vi "Start.vi"(8 "error in (no error)":errorcluster, 10 "Message in":refnum<class "StartMessage.lvclass">, 11 "DAQMH121119OrcaFlash in":refnum<class "DAQOrcaFlash.lvclass">) -> (0 "error out":errorcluster, 3 "DAQMH121119OrcaFlash out":refnum<class "DAQOrcaFlash.lvclass">)   [LabVIEW 2012, in "DAQOrcaFlash.lvclass"]
doc: "This member function is called when the statemachine in the run.vi receives an 'start' command. It relays the message to all observers of the component.\n\nOverride this member function in your derived class if you need additional start functionality (but don't forget to call the parent method)."
uses:
  DAQOrcaFlash.lvclass
  <vilib>/Distrio/Murmex/StartMessage/StartMessage.lvclass
  <vilib>/Distrio/Murmex/Murmex/Murmex.lvclass
  DAQOrcaFlash.lvclass/DAQOrcaFlash.ctl
  <vilib>/Distrio/Murmex/ProceedMessage/ProceedMessage.lvclass
  imaging_mode.ctl
panel:
  # "This method is called when the START\ntrigger is sent. \n\nOverride this method when your component needs to\nrespond to this trigger. \n\nCall parent for proper implementation"
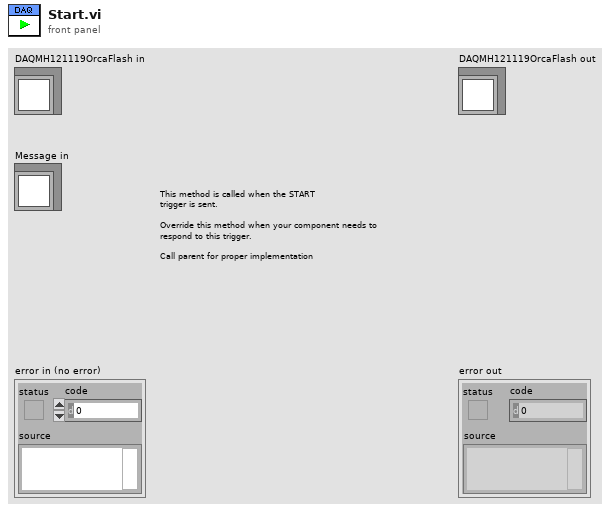
[diagram p1: front panel]
types:
  T1 = cluster{"Mode":u32, "Polarity":u32, "Period":dbl, "Delay":dbl}
  T2 = typedef "DAQOrcaFlash.lvclass/imaging_mode.ctl" = enum16{"focus mode", "single sweep"}
  T3 = typedef "Murmex.lvlib/StartMessage.lvclass/run mode enum.ctl" = enum16{"infinite", "finite"}
  T4 = typedef "IMAQ Image.ctl" = refnum<image>
  T5 = cluster{"width":u32, "height":u32, "datatype":u32}
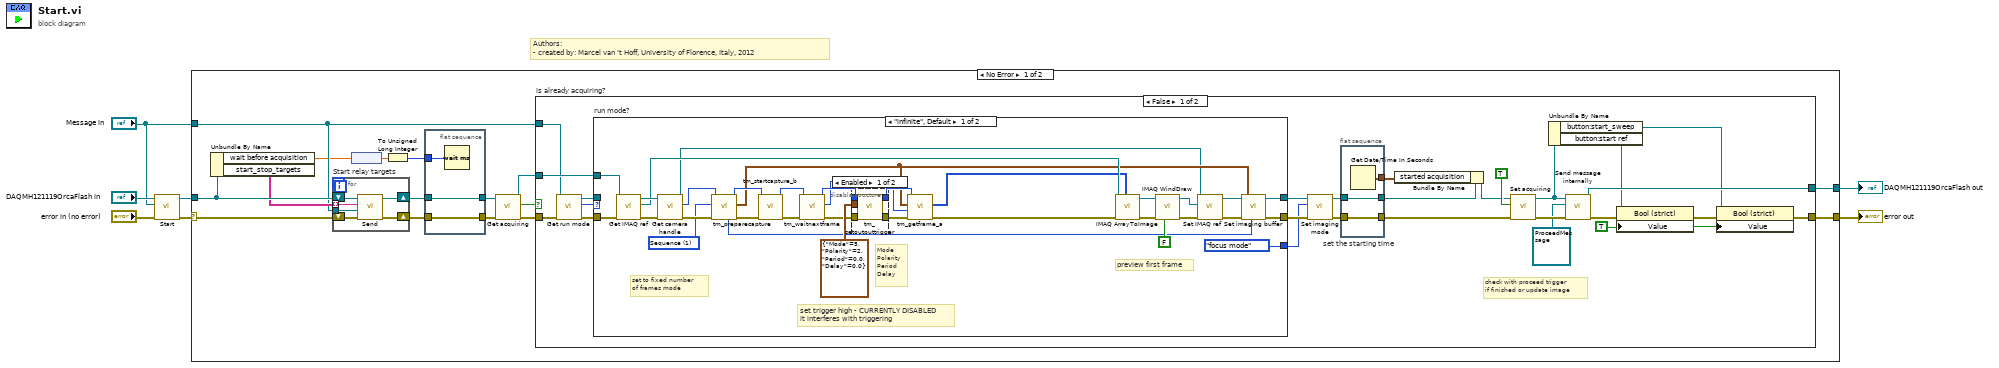
[diagram p0: block diagram]
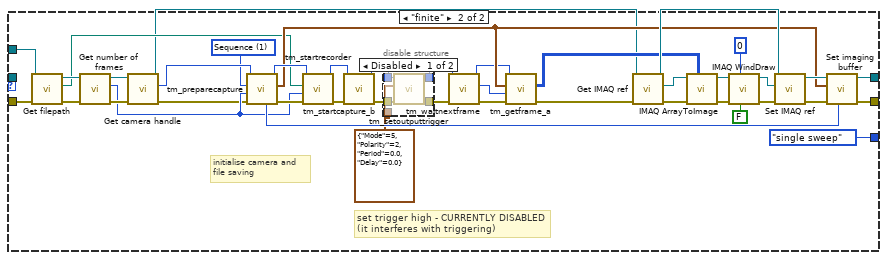
[diagram p3: hidden frame]
diagram:
  # "Authors: \n- created by: Marcel van 't Hoff, University of Florence, Italy, 2012"
  n1 = call-parent "Start.vi"("error in (no error)"="error in (no error)", "Message in"="Message in", "Murmex in"="DAQMH121119OrcaFlash in") -> ("error out"=w3:errorcluster, "Murmex out"=w4:refnum<class "DAQOrcaFlash.lvclass">)  [unwired: 7 in]
  n2 = case shown="No Error" w3 {
    selector: w3 -> [w16 w154]
    tunnel: [w23 w154] -> w2
    tunnel: [w22 w153] -> w7
    tunnel: w4 -> [w18 w153]
    tunnel: "Message in" -> [w11 _]
    frame No Error {
      n3 = Unbundle By Name(w18) -> ("wait before acquisition"=w10:dbl[unit], "start_stop_targets"=w17:string[])
      n4 = for "Start relay targets" {
        shift-right: [w32] -> w14
        shift-left: w16 -> [w31]
        tunnel: w11 -> [w29]
        tunnel: w17 -> [w28] mode=indexing
        shift-right: [w27] -> w12
        shift-left: w18 -> [w30]
        n5 = call <vilib>:"Send.vi"("error in (no error)"=w31, "Message"=w29, "recipient"=w28, "Murmex in"=w30) -> ("error out"=w32:errorcluster, "Murmex out"=w27:refnum<class "DAQOrcaFlash.lvclass">)  [unwired: 6 in]
      }
      n6 = node(w10) -> (w9:dbl)
      n7 = To Unsigned Long Integer(number=w9) -> (unsigned 32bit integer=w8:u32)
      n8 = flat-sequence {
        tunnel: [w26] -> w15
        tunnel: w14 -> [w26]
        tunnel: [w25] -> w13
        tunnel: w12 -> [w25]
        tunnel: w8 -> [w24]
        frame #0 {
          n9 = Wait (ms)(milliseconds to wait=w24) -> ()  [unwired: 1 out]
        }
      }
      n10 = call "Get acquiring.vi"("error in (no error)"=w15, "DAQMH121119OrcaFlash in"=w13) -> ("error out"=w20:errorcluster, "is acquiring?"=w19:bool, "DAQMH121119OrcaFlash out"=w21:refnum<class "DAQOrcaFlash.lvclass">)  [unwired: 7 in]
      n11 = case "is already acquiring?" shown="False" w19 {
        tunnel: [w46 w152] -> w23
        tunnel: [w57 w151] -> w22
        tunnel: w21 -> [w44 w151]
        tunnel: w20 -> [w37 w152]
        tunnel: w11 -> [w33 _]
        frame False {
          w48 = TRUE ("Value")
          # "check with proceed trigger\nif finished or update image"
          n12 = call <vilib>:"Get run mode.vi"("error in (no error)"=w37, "StartMessage in"=w33) -> ("error out"=w36:errorcluster, "run mode"=w35:T3, "StartMessage out"=w34:refnum<class "StartMessage.lvclass">)  [unwired: 7 in]
          n13 = case "run mode?" shown="\"infinite\", Default" w35 {
            tunnel: w36 -> [w92 w109]
            tunnel: [w89 w133] -> w56
            tunnel: [w90 w134] -> w42
            tunnel: w44 -> [w94 w107]
            tunnel: [imaging_mode."focus mode" ("imaging mode") imaging_mode."single sweep" ("imaging mode")] -> w40
            tunnel: w34 -> [_ _]
            frame "infinite", Default {
              w78 = 1 items=["Snap", "Sequence"] ("Capture mode")
              # "Mode\nPolarity\nPeriod\nDelay"
              # "set trigger high - CURRENTLY DISABLED\nit interferes with triggering"
              # "preview first frame"
              # "set to fixed number\nof frames mode"
              n14 = call "Get IMAQ ref.vi"("error in (no error)"=w92, "DAQMH121119OrcaFlash in"=w94) -> ("error out"=w91:errorcluster, "IMAQ reference"=w69:T4, "DAQMH121119OrcaFlash out"=w93:refnum<class "DAQOrcaFlash.lvclass">)  [unwired: 7 in]
              n15 = call "Get camera handle.vi"("error in (no error)"=w91, "DAQMH121119OrcaFlash in"=w93) -> ("error out"=w80:errorcluster, "cam handle"=w77:u32, "DAQMH121119OrcaFlash out"=w62:refnum<class "DAQOrcaFlash.lvclass">)  [unwired: 7 in]
              n16 = call <userlib>:"tm_preparecapture.vi"("error in (no error)"=w80, "Capture mode"=w78, "Handle in"=w77) -> ("error out"=w79:errorcluster, "Buffer"=w67:T5, "Handle out"=w76:u32, "Image type"=w66:u32)  [unwired: 5 in]
              n17 = call <userlib>:"tm_startcapture_b.vi"("error in (no error)"=w79, "Handle in"=w76) -> ("error out"=w74:errorcluster, "Handle out"=w75:u32)  [unwired: 8 in]
              n18 = call <userlib>:"tm_waitnextframe.vi"("error in (no error)"=w74, "Handle in"=w75) -> ("error out"=w81:errorcluster, "Frame Index"=w71:i32, "Handle out"=w82:u32)  [unwired: 6 in, 1 out]
              n19 = disable-structure shown="Enabled" {
                disable-tunnel: T1 {"Mode"=5, "Polarity"=2, "Period"=0.0, "Delay"=0.0} ("Parameters") -> [w99 _]
                disable-tunnel: w82 -> [w98 w100]
                disable-tunnel: w81 -> [w97 w101]
                disable-tunnel: [w96 w101] -> w73
                disable-tunnel: [w95 w100] -> w72
                frame Enabled {
                  n20 = call <userlib>:"tm_setoutputtrigger.vi"("error in (no error)"=w97, "Parameters"=w99, "Handle in"=w98) -> ("error out"=w96:errorcluster, "Handle out"=w95:u32)  [unwired: 7 in]
                }
                frame Disabled {
                }
              }
              n21 = call <userlib>:"tm_getframe_a.vi"("error in (no error)"=w73, "Frame Index"=w71, "Buffer"=w67, "Handle in"=w72) -> ("error out"=w63:errorcluster, "Data 16"=w65:u16[][])  [unwired: 3 in, 3 out]
              n22 = call "IMAQ ArrayToImage"("Image Pixels (U16)"=w65, "error in (no error)"=w63, "Image"=w69) -> ("error out"=w70:errorcluster, "Image Out"=w68:T4)  [unwired: 7 in]
              n23 = call "IMAQ WindDraw"("Resize to Image Size? (Y)"=FALSE, "error in (no error)"=w70, "Image"=w68) -> ("error out"=w85:errorcluster, "Image Out (duplicate)"=w64:T4)  [unwired: 7 in]
              n24 = call "Set IMAQ ref.vi"("error in (no error)"=w85, "IMAQ reference"=w64, "DAQMH121119OrcaFlash in"=w62) -> ("error out"=w86:errorcluster, "DAQMH121119OrcaFlash out"=w87:refnum<class "DAQOrcaFlash.lvclass">)  [unwired: 7 in]
              n25 = call "Set imaging buffer.vi"("Image type"=w66, "error in (no error)"=w86, "Buffer"=w67, "DAQMH121119OrcaFlash in"=w87) -> ("error out"=w89:errorcluster, "DAQMH121119OrcaFlash out"=w90:refnum<class "DAQOrcaFlash.lvclass">)  [unwired: 6 in]
            }
            frame "finite" {
              w138 = 1 items=["Snap", "Sequence"] ("Capture mode")
              # "set trigger high - CURRENTLY DISABLED\n(it interferes with triggering)"
              # "initialise camera and\nfile saving"
              n26 = call "Get filepath.vi"("error in (no error)"=w109, "DAQOrcaFlash in"=w107) -> ("error out"=w108:errorcluster, "filepath out"=w105:path, "DAQOrcaFlash out"=w106:refnum<class "DAQOrcaFlash.lvclass">)  [unwired: 7 in]
              n27 = call "Get number of frames.vi"("error in (no error)"=w108, "DAQMH121119OrcaFlash in"=w106) -> ("error out"=w143:errorcluster, "no. of frames"=w104:i32, "DAQMH121119OrcaFlash out"=w142:refnum<class "DAQOrcaFlash.lvclass">)  [unwired: 7 in]
              n28 = call "Get camera handle.vi"("error in (no error)"=w143, "DAQMH121119OrcaFlash in"=w142) -> ("error out"=w103:errorcluster, "cam handle"=w141:u32, "DAQMH121119OrcaFlash out"=w102:refnum<class "DAQOrcaFlash.lvclass">)  [unwired: 7 in]
              n29 = call <userlib>:"tm_preparecapture.vi"("error in (no error)"=w103, "Frames"=w104, "Capture mode"=w138, "Handle in"=w141) -> ("error out"=w139:errorcluster, "Buffer"=w124:T5, "Handle out"=w140:u32, "Image type"=w131:u32)  [unwired: 4 in]
              n30 = call <userlib>:"tm_startrecorder.vi"("error in (no error)"=w139, "frames"=w104, "File"=w105, "Handle in"=w140) -> ("error out"=w122:errorcluster, "Handle out"=w123:u32)  [unwired: 6 in]
              n31 = call <userlib>:"tm_startcapture_b.vi"("error in (no error)"=w122, "Handle in"=w123) -> ("error out"=w111:errorcluster, "Handle out"=w113:u32)  [unwired: 8 in]
              n32 = disable-structure shown="Disabled" {
                disable-tunnel: T1 {"Mode"=5, "Polarity"=2, "Period"=0.0, "Delay"=0.0} ("Parameters") -> [w148 _]
                disable-tunnel: w113 -> [w147 w150]
                disable-tunnel: [w146 w150] -> w112
                disable-tunnel: w111 -> [w145 w149]
                disable-tunnel: [w144 w149] -> w110
                frame Disabled {
                  n33 = call <userlib>:"tm_setoutputtrigger.vi"("error in (no error)"=w145, "Parameters"=w148, "Handle in"=w147) -> ("error out"=w144:errorcluster, "Handle out"=w146:u32)  [unwired: 7 in]
                }
                frame Enabled {
                }
              }
              n34 = call <userlib>:"tm_waitnextframe.vi"("error in (no error)"=w110, "Handle in"=w112) -> ("error out"=w130:errorcluster, "Frame Index"=w128:i32, "Handle out"=w115:u32)  [unwired: 6 in, 1 out]
              n35 = call <userlib>:"tm_getframe_a.vi"("error in (no error)"=w130, "Frame Index"=w128, "Buffer"=w124, "Handle in"=w115) -> ("error out"=w129:errorcluster, "Data 16"=w127:u16[][])  [unwired: 3 in, 3 out]
              n36 = call "Get IMAQ ref.vi"("error in (no error)"=w129, "DAQMH121119OrcaFlash in"=w102) -> ("error out"=w125:errorcluster, "IMAQ reference"=w126:T4, "DAQMH121119OrcaFlash out"=w137:refnum<class "DAQOrcaFlash.lvclass">)  [unwired: 7 in]
              n37 = call "IMAQ ArrayToImage"("Image Pixels (U16)"=w127, "error in (no error)"=w125, "Image"=w126) -> ("error out"=w120:errorcluster, "Image Out"=w121:T4)  [unwired: 7 in]
              n38 = call "IMAQ WindDraw"("Resize to Image Size? (Y)"=FALSE, "Window Number (0...15)"=0, "error in (no error)"=w120, "Image"=w121) -> ("error out"=w119:errorcluster, "Image Out (duplicate)"=w118:T4)  [unwired: 6 in]
              n39 = call "Set IMAQ ref.vi"("error in (no error)"=w119, "IMAQ reference"=w118, "DAQMH121119OrcaFlash in"=w137) -> ("error out"=w136:errorcluster, "DAQMH121119OrcaFlash out"=w135:refnum<class "DAQOrcaFlash.lvclass">)  [unwired: 7 in]
              n40 = call "Set imaging buffer.vi"("Image type"=w131, "error in (no error)"=w136, "Buffer"=w124, "DAQMH121119OrcaFlash in"=w135) -> ("error out"=w133:errorcluster, "DAQMH121119OrcaFlash out"=w134:refnum<class "DAQOrcaFlash.lvclass">)  [unwired: 6 in]
            }
          }
          n41 = call "Set imaging mode.vi"("error in (no error)"=w56, "imaging mode"=w40, "DAQMH121119OrcaFlash in"=w42) -> ("error out"=w43:errorcluster, "DAQMH121119OrcaFlash out"=w41:refnum<class "DAQOrcaFlash.lvclass">)  [unwired: 7 in]
          n42 = flat-sequence "set the starting time" {
            tunnel: [w61] -> w52
            tunnel: w41 -> [w61]
            tunnel: w43 -> [w60]
            tunnel: [w60] -> w55
            tunnel: [w59] -> w54
            frame #0 {
              n43 = Get Date/Time In Seconds() -> (seconds since 1Jan1904=w59:timestamp)
            }
          }
          n44 = Bundle By Name(cluster=w52, "started acquisition"=w54) -> (w53:refnum<class "DAQOrcaFlash.lvclass">)
          n45 = call "Set acquiring.vi"("error in (no error)"=w55, "is acquiring?"=TRUE, "DAQMH121119OrcaFlash in"=w53) -> ("error out"=w39:errorcluster, "DAQMH121119OrcaFlash out"=w51:refnum<class "DAQOrcaFlash.lvclass">)  [unwired: 7 in]
          n46 = Unbundle By Name(w51) -> ("button:start_sweep"=w45:refnum<vi>, "button:start ref"=w50:refnum<vi>)
          n47 = call <vilib>:"Send message internally.vi"("error in (no error)"=w39, "Message"=refnum<class "ProceedMessage.lvclass"> refnum ("ProceedMessage"), "Murmex in"=w51) -> ("error out"=w49:errorcluster, "Murmex out"=w57:refnum<class "DAQOrcaFlash.lvclass">)  [unwired: 7 in]
          n48 = property class="Bool (strict)"(reference=w50, error in=w49, "Value"=w48) -> (error out=w47:errorcluster)  [unwired: 1 out]
          n49 = property class="Bool (strict)"(reference=w45, error in=w47, "Value"=w48) -> (error out=w46:errorcluster)  [unwired: 1 out]
        }
        frame True {
          # "Skip double start trigger events"
        }
      }
    }
    frame Error {
    }
  }
  "DAQMH121119OrcaFlash out" <- w7
  "error out" <- w2
